vi "Test_AWG_5421_Standalone.vi"(8 "error in (no error)":errorcluster, 10 "AWG 5421 Inputs":T1={"Resource Name"="AWG_5421", "Sample Rate"=10000000.0, "Trigger Type"=2, "Trigger Source"="PFI0", "Waveform Gain"=0.31, "Digital Filter ON"=TRUE} {"Sample Rate" format="%.2p"; "Trigger Type" items=["None", "Software Edge", "Digital Edge", "Digital Level"]}, 11 "Use Software Trigger":bool=TRUE) -> (0 "error out":errorcluster)   [LabVIEW 2018]
doc: "This VI inits a waveform generation session for AWG-5421. This is a basic example that shows how to setup the board in order to generate waveforms according to a script. \nBy default this configuration uses one channel CH0, and one script trigger ScriptTrigger0. The ScriptTrigger0 is waiting for an external trigger : i.e. a digital Edge on pin PFI 0 by default.\n\nThere are various options for the script to be used. Consult the Script control help for more information on configuring the example for specific scripts."
uses:
  controls/AWG_5421_Inputs.ctl
  <instrlib>/niFgen/niFgen.llb/niFgen_ctl Trigger Source Values (Ring).ctl
  <instrlib>/niFgen/niFgen.llb/niFgen Output Mode.ctl
  <instrlib>/niFgen/niFgen.llb/niFgen_ctl Sample Clock Source Values (Ring).ctl
  <instrlib>/niFgen/niFgen.llb/niFgen_ctl Trigger Script - trigID Values (Ring).ctl
  <instrlib>/niFgen/niFgen.llb/niFgen_ctl Trigger DigEdge - Edge Values (Ring).ctl
  <instrlib>/niFgen/niFgen.llb/niFgen Configure Software Edge Script Trigger.vi
  <instrlib>/niFgen/niFgen.llb/niFgen Configure Digital Edge Script Trigger.vi
  <instrlib>/niFgen/niFgen.llb/niFgen Write Named Waveform (DBL).vi
panel:
  in  "Amplitude":dbl=2.0 caption="Amplitude (Pk-Pk)" format="%.4f"
  in  "Script 2 (NOT USED)":string="script myScript0\n    wait until scriptTrigger0\n    Generate Sinus250to250a100dur800fs10\nend script"
  out "taille(s)":i32
  out "Graphe":dbl[](graph)
  in  "Script":string="script myScript0\n    wait until scriptTrigger0\n    repeat 1000\n       Generate E1Swift0p5f150p0to550p0a70d1200fs20\n    end repeat\nend script"
  in  "Send Software Trigger":bool
  # "Si Use SW Trigger pas utilisé, connecter HSDIO et envoyer avec NI-MAX une impulsion en sortie de HSDIO (pin n°6). Si utilisé, clic sur Send SW Trigger"
  # "ATTENTION\nModifier Sample Rate\nen fonction de la forme\nqui est codee en dur dans le\ndiagramme !!!"
  # "ATTENTION\nsi wait until scriptTrigger0 dans le\nscript alors obligatoirement\nattente d'un trigger (soft ou hard)"
  # "ATTENTION\nsi AUCUN wait until scriptTrigger0\ndans le script alors generation\nimmediate de la waveform"
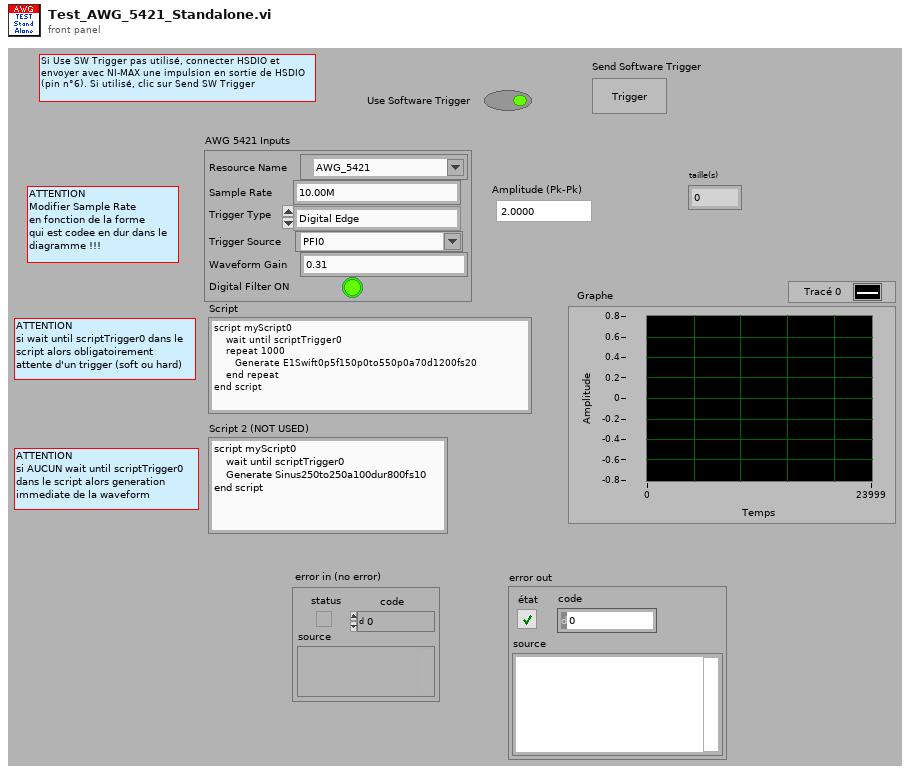
[diagram p1: front panel]
types:
  T1 = typedef "AWG_5421_Inputs.ctl" = cluster{"Resource Name":refnum<k15>, "Sample Rate":dbl, "Trigger Type":u16, "Trigger Source":T2, "Waveform Gain":dbl, "Digital Filter ON":bool}
  T2 = typedef "niFgen_ctl Trigger Source Values (Ring).ctl" = string
  T3 = typedef "niFgen_ctl Sample Clock Source Values (Ring).ctl" = string
  T4 = typedef "niFgen_ctl Trigger Script - trigID Values (Ring).ctl" = string
  T5 = enum16{"big-endian, network order", "native, host order", "little-endian"}
  T6 = enum16{"open", "replace", "create", "open or create", "replace or create", "replace or create with confirmation"}
  T7 = typedef "niFgen Output Mode.ctl" = u32
  T8 = typedef "niFgen_ctl Trigger DigEdge - Edge Values (Ring).ctl" = i32
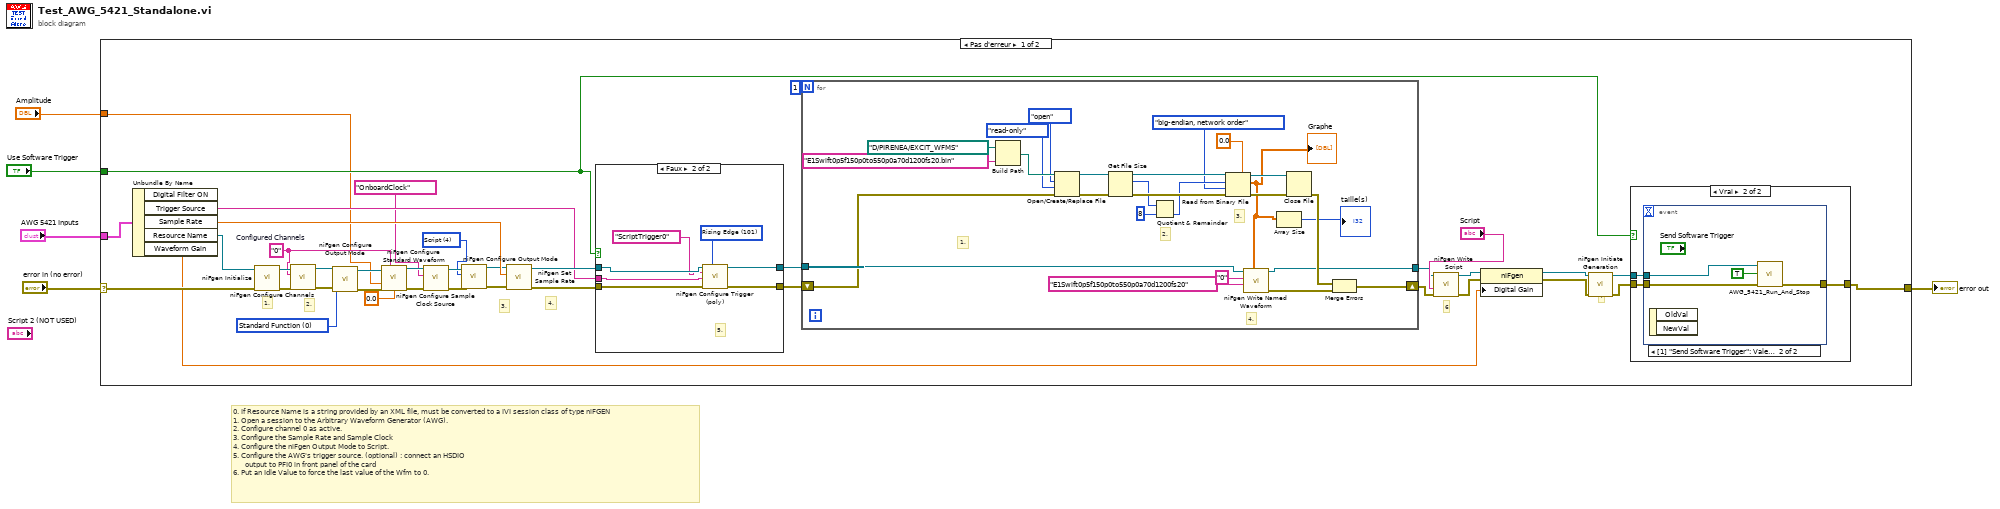
[diagram p0: block diagram]
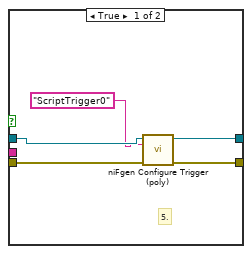
[diagram p2: hidden frame]
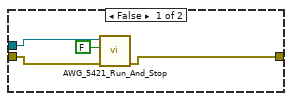
[diagram p3: hidden frame]
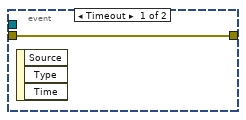
[diagram p4: hidden frame]
diagram:
  # "0. If Resource Name is a string provided by an XML file, must be converted to a IVI session class of type niFGEN\n1. Open a session to the Arbitrary Waveform Generator (AWG).\n2. Configure channel 0 as active. \n3. Configure the Sample Rate and Sample Clock\n4. Configure the niFgen Output Mode to Script.\n5. Configure the AWG's trigger source. (optional) : connect an HSDIO\n      output to PFI0 in front panel of the card \n6. Put an Idle Value to force the last value of the Wfm to 0."
  n1 = case shown="Pas d'erreur" "error in (no error)" {
    selector: "error in (no error)" -> [w37 w96]
    tunnel: [w27 w96] -> w5
    tunnel: "AWG 5421 Inputs" -> [w45 _]
    tunnel: "Use Software Trigger" -> [w28 _]
    tunnel: "Amplitude" -> [w7 _]
    frame No Error {
      w19 = T7 0 items=["Standard Function", "Frequency List", "Arbitrary Waveform", "Arbitrary Sequence", "Script"] ("Output Mode (default: 0=Standard Function)")
      w16 = "0"  # Configured Channels
      w10 = T7 4 items=["Standard Function", "Frequency List", "Arbitrary Waveform", "Arbitrary Sequence", "Script"] ("Output Mode")
      # "6"
      # "7"
      # "4."
      # "3."
      # "2."
      # "1."
      n2 = Unbundle By Name(w45) -> ("Trigger Source"=w39:T2, "Sample Rate"=w42:dbl, "Resource Name"=w38:refnum<k15>, "Waveform Gain"=w22:dbl)  [unwired: 1 out]
      n3 = call <instrlib>:"niFgen Initialize.vi"("error in (no error)"=w37, "Resource Name"=w38) -> ("error out"=w40:errorcluster, "Instrument Handle Out"=w41:refnum<k15>)  [unwired: 8 in]
      n4 = call <instrlib>:"niFgen Configure Channels.vi"("error in (no error)"=w40, "Channels"=w16, "Instrument Handle"=w41) -> ("error out"=w20:errorcluster, "Instrument Handle Out"=w21:refnum<k15>)  [unwired: 7 in]
      n5 = call <instrlib>:"niFgen Configure Output Mode.vi"("error in (no error)"=w20, "Output Mode (default: 0=Standard Function)"=w19, "Instrument Handle"=w21) -> ("error out"=w17:errorcluster, "Instrument Handle Out"=w18:refnum<k15>)  [unwired: 6 in]
      n6 = call <instrlib>:"niFgen Configure Standard Waveform.vi"("Instrument Handle"=w18, "Channel Name"=w16, "Amplitude"=w7, "error in (no error)"=w17, "DC Offset"=0.0) -> ("Instrument Handle Out"=w14:refnum<k15>, "error out"=w15:errorcluster)  [unwired: 9 in]
      n7 = call <instrlib>:"niFgen Configure Sample Clock Source.vi"("error in (no error)"=w15, "Source (Onboard Clock)"=T3 "OnboardClock", "Instrument Handle"=w14) -> ("error out"=w12:errorcluster, "Instrument Handle Out"=w11:refnum<k15>)  [unwired: 7 in]
      n8 = call <instrlib>:"niFgen Configure Output Mode.vi"("error in (no error)"=w12, "Output Mode (default: 0=Standard Function)"=w10, "Instrument Handle"=w11) -> ("error out"=w8:errorcluster, "Instrument Handle Out"=w9:refnum<k15>)  [unwired: 6 in]
      n9 = call <instrlib>:"niFgen Set Sample Rate.vi"("error in (no error)"=w8, "Sample Rate (Samp/s)"=w42, "Instrument Handle"=w9) -> ("error out"=w43:errorcluster, "Instrument Handle Out"=w44:refnum<k15>)  [unwired: 7 in]
      n10 = case shown="Faux" w28 {
        tunnel: w44 -> [w50 w57]
        tunnel: w43 -> [w49 w56]
        tunnel: w39 -> [_ w55]
        tunnel: [w48 w54] -> w35
        tunnel: [w47 w53] -> w34
        frame True {
          # "5."
          n11 = call-poly <instrlib>:"niFgen Configure Trigger (poly).vi"("error in (no error)"=w49, "Trigger ID (Script Trigger 0)"=T4 "ScriptTrigger0", "Instrument Handle"=w50) -> ("error out"=w48:errorcluster, "Instrument Handle Out"=w47:refnum<k15>)  [unwired: 7 in]
        }
        frame False {
          w51 = T8 101 items=["Rising Edge"=101, "Falling Edge"=102] ("Edge (Rising)")
          # "5."
          n12 = call-poly <instrlib>:"niFgen Configure Trigger (poly).vi"("Edge (Rising)"=w51, "error in (no error)"=w56, "Source"=w55, "Trigger ID (Script Trigger 0)"=T4 "ScriptTrigger0", "Instrument Handle"=w57) -> ("error out"=w54:errorcluster, "Instrument Handle Out"=w53:refnum<k15>)  [unwired: 5 in]
        }
      }
      n13 = for {
        N: 1 -> [_]
        shift-right: [w69] -> w31
        shift-left: w35 -> [w60]
        tunnel: [w67] -> w32
        tunnel: w34 -> [w64]
        # "4."
        # "3."
        # "2."
        # "1."
        n14 = Build Path(base path=path "D:/PIRENEA/EXCIT_WFMS" ("chemin de base"), name or relative path="E1Swift0p5f150p0to550p0a70d1200fs20.bin" ("nom ou chemin relatif")) -> (appended path=w81:path)
        n15 = Open/Create/Replace File(file path (use dialog)=w81, error in=w60, operation (0:open)=T6."open", access (0:read/write)=enum16{"read/write", "read-only", "write-only"}."read-only") -> (refnum out=w83:refnum<file>, error out=w82:errorcluster)  [unwired: 2 in, 1 out]
        n16 = Get File Size(file=w83, error in=w82) -> (refnum out=w77:refnum<file>, size (in bytes)=w65:i64, 0:w75:errorcluster)
        n17 = Quotient & Remainder(x=w65, y=i64 8 ("type size (bytes)")) -> (floor(x/y)=w73:i64)  [unwired: 1 out]
        n18 = Read from Binary File(5:0.0 ("data type"), 8:w75, 9:T5."big-endian, network order" ("ordre des octets (0 : big-Endian, network order)"), 10:w73, 11:w77) -> (0:w74:errorcluster, 2:w58:dbl[], 3:w76:refnum<file>)  [unwired: 1 in, 1 out]
        "Graphe" <- w58
        n19 = call-poly <instrlib>:"niFgen Write Named Waveform.vi"("Waveform Data"=w58, "Waveform Name"="E1Swift0p5f150p0to550p0a70d1200fs20", "Channel Name"="0", "Instrument Handle"=w64) -> ("error out"=w68:errorcluster, "Instrument Handle Out"=w67:refnum<k15>)  [unwired: 5 in, 1 out]
        n20 = Array Size(array=w58) -> (size(s)=→"taille(s)":i32)
        n21 = Close File(refnum=w76, error in=w74) -> (error out=w70:errorcluster)  [unwired: 1 out]
        n22 = Merge Errors(w70, w68) -> (w69:errorcluster)
      }
      n23 = call <instrlib>:"niFgen Write Script.vi"("error in (no error)"=w31, "Script"="Script", "Instrument Handle"=w32) -> ("error out"=w25:errorcluster, "Instrument Handle Out"=w26:refnum<k15>)  [unwired: 7 in]
      n24 = property class="niFgen"(reference=w26, error in=w25, "Digital Gain"=w22) -> (reference out=w24:refnum<k15>, error out=w23:errorcluster)
      n25 = call <instrlib>:"niFgen Initiate Generation.vi"("error in (no error)"=w23, "Instrument Handle"=w24) -> ("error out"=w29:errorcluster, "Instrument Handle Out"=w30:refnum<k15>)  [unwired: 8 in]
      n26 = case shown="Vrai" w28 {
        tunnel: w30 -> [w87 w90]
        tunnel: w29 -> [w86 w89]
        tunnel: [w84 w88] -> w27
        frame False {
          n27 = call "AWG_5421_Run_And_Stop.vi"("error  in"=w86, "Use Software trigger"=FALSE, "instrument handle in"=w87) -> ("error out"=w84:errorcluster)  [unwired: 8 in]
        }
        frame True {
          n28 = event shown="[1] \"Send Software Trigger\": Valeur changée" {
            selector: _ -> [_ _]
            dyn-events: _ -> [_ _]
            timeout: _ -> [_ _]
            tunnel: [w91 w95] -> w88
            tunnel: w90 -> [_ w94]
            tunnel: w89 -> [w91 w93]
            event Timeout {
              n29 = event-data() -> ()  [unwired: 1 in, 3 out]
            }
            event "Send Software Trigger": Value Change {
              n30 = event-data() -> ()  [unwired: 1 in, 2 out]
              n31 = call "AWG_5421_Run_And_Stop.vi"("error  in"=w93, "Use Software trigger"=TRUE, "instrument handle in"=w94) -> ("error out"=w95:errorcluster)  [unwired: 8 in]
            }
          }
        }
      }
    }
    frame Error {
    }
  }
  "error out" <- w5
